vi "MeasurementType.Create.IPCore.vi"(8 "error in (no error)":errorcluster, 9 "Name":string, 11 "Parent":T1 format="%.0x") -> (0 "error out":errorcluster, 1 "Child Name":string, 2 "Child":T1 format="%.0x", 3 "Parent":T1 format="%.0x")   [LabVIEW 2015, in "Fuel Injector Analysis Addon System Explorer.lvlib"]
uses:
  <vilib>/NI Veristand/Custom Device API/Custom Device Item Ref.ctl
  Shared/Constants.vi
  <vilib>/NI Veristand/Custom Device Tools/Custom Device Utility Library/NI VeriStand - Search for Item by Name.vi
  Fuel Injector Analysis Addon System Explorer.lvlib
  <vilib>/NI Veristand/Custom Device Tools/Custom Device Utility Library/Custom Device Utility Library.lvlib
  <vilib>/NI VeriStand/Custom Device API/Custom Device API.lvlib
  Shared/Fuel Injector Analysis Addon Shared.lvlib
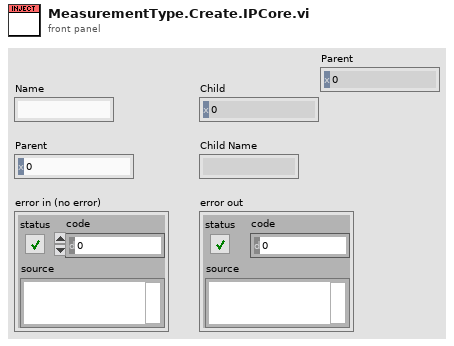
[diagram p1: front panel]
types:
  T1 = typedef "Custom Device API.lvlib/Custom Device Item Ref.ctl" = u64
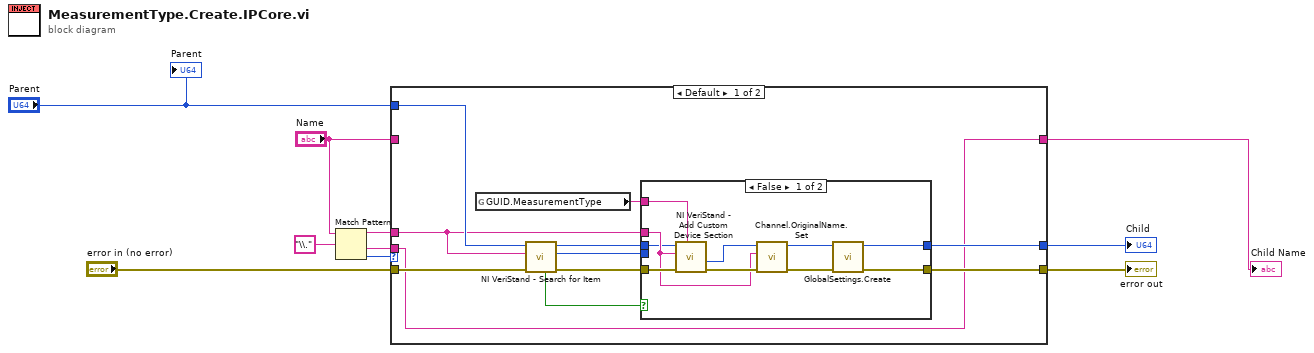
[diagram p0: block diagram]
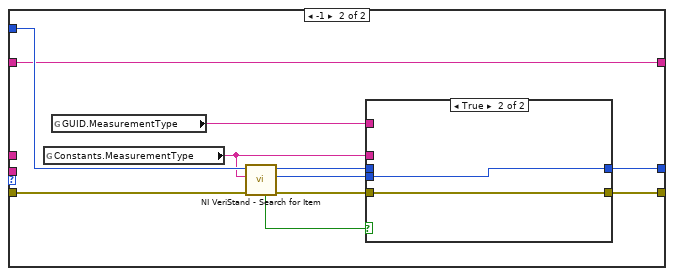
[diagram p3: hidden frame]
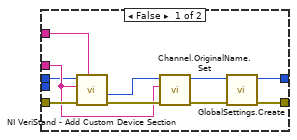
[diagram p4: hidden frame]
diagram:
  n1 = Match Pattern(string="Name", regular expression="\\.") -> (before substring=w4:string, after substring=w10:string, offset past match=w2:i32)  [unwired: 1 in, 1 out]
  n2 = case shown="Default" w2 {
    tunnel: "error in (no error)" -> [w21 w41]
    tunnel: w4 -> [w12 _]
    tunnel: "Parent" -> [w20 w38]
    tunnel: [w16 w40] -> w5
    tunnel: [w15 w39] -> w7
    tunnel: [w11 w35] -> w8
    tunnel: "Name" -> [_ w35]
    tunnel: w10 -> [w11 _]
    frame Default {
      n3 = global read "Constants.vi" "GUID.MeasurementType"() -> (w14:string)
      n4 = call-poly <vilib>:"NI VeriStand - Search for Item.vi"("error in"=w21, "Item Name"=w12, "Section Ref in"=w20) -> ("error out"=w19:errorcluster, "Item Ref"=w18:T1, "Section Ref out"=w13:T1, "Found"=w17:bool)  [unwired: 5 in]
      n5 = case shown="False" w17 {
        tunnel: w19 -> [w31 w33]
        tunnel: w18 -> [_ w32]
        tunnel: [w23 w33] -> w16
        tunnel: [w24 w32] -> w15
        tunnel: w12 -> [w27 _]
        tunnel: w14 -> [w30 _]
        tunnel: w13 -> [w22 _]
        frame False {
          n6 = call <vilib>:"NI VeriStand - Add Custom Device Section.vi"("GUID (Default Section)"=w30, "error in (no error)"=w31, "Section Name"=w27, "Parent Ref in"=w22) -> ("error out"=w29:errorcluster, "Section Ptr"=w28:T1)  [unwired: 4 in, 2 out]
          n7 = call "Channel.OriginalName.Set.vi"("error in (no error)"=w29, "Constants.Channel Name"=w27, "Ref"=w28) -> ("error out"=w26:errorcluster, "Ref out"=w25:T1)  [unwired: 7 in]
          n8 = call "GlobalSettings.Create.vi"("error in (no error)"=w26, "Device Item Ref in"=w25) -> ("error out"=w23:errorcluster, "Parent Ref out"=w24:T1)  [unwired: 8 in]
        }
        frame True {
        }
      }
    }
    frame -1 {
      n9 = global read "Constants.vi" "Constants.MeasurementType"() -> (w36:string)
      n10 = global read "Constants.vi" "GUID.MeasurementType"() -> (w37:string)
      n11 = call-poly <vilib>:"NI VeriStand - Search for Item.vi"("error in"=w41, "Item Name"=w36, "Section Ref in"=w38) -> ("error out"=w44:errorcluster, "Item Ref"=w43:T1, "Section Ref out"=w34:T1, "Found"=w42:bool)  [unwired: 5 in]
      n12 = case shown="True" w42 {
        tunnel: w44 -> [w54 w56]
        tunnel: w43 -> [_ w55]
        tunnel: [w46 w56] -> w40
        tunnel: [w47 w55] -> w39
        tunnel: w36 -> [w50 _]
        tunnel: w37 -> [w53 _]
        tunnel: w34 -> [w45 _]
        frame False {
          n13 = call <vilib>:"NI VeriStand - Add Custom Device Section.vi"("GUID (Default Section)"=w53, "error in (no error)"=w54, "Section Name"=w50, "Parent Ref in"=w45) -> ("error out"=w51:errorcluster, "Section Ptr"=w52:T1)  [unwired: 4 in, 2 out]
          n14 = call "Channel.OriginalName.Set.vi"("error in (no error)"=w51, "Constants.Channel Name"=w50, "Ref"=w52) -> ("error out"=w49:errorcluster, "Ref out"=w48:T1)  [unwired: 7 in]
          n15 = call "GlobalSettings.Create.vi"("error in (no error)"=w49, "Device Item Ref in"=w48) -> ("error out"=w46:errorcluster, "Parent Ref out"=w47:T1)  [unwired: 8 in]
        }
        frame True {
        }
      }
    }
  }
  "Child Name" <- w8
  "Child" <- w7
  "error out" <- w5
  "Parent" <- "Parent"
